vi "New DAQ Rack AI Read.vi"(8 "Rack Version":T2, 9 "Cal Unit":T3, 10 "Channel to Cal":T1, 11 "Chassis":tag) -> (0 "Lost Connection":bool, 2 "Available?":bool, 3 "Data":dbl format="%0.2f")   [LabVIEW 2013]
uses:
  Type Defs/Units Type Def (DAQ Rack).ctl
  Type Defs/Rack Version Type Def.ctl
  Type Defs/New Channel Type Def (RIO).ctl
  Type Defs/TCP Data Stream Mode (PC).ctl
  <vilib>/DAQmx/read.llb/DAQmx Read (Analog DBL 1Chan 1Samp).vi
  <vilib>/DAQmx/read.llb/DAQmx Read (Analog 1D DBL 1Chan NSamp).vi
  <vilib>/DAQmx/create/channels.llb/DAQmx Create Channel (AI-Voltage-Basic).vi
  <vilib>/DAQmx/miscellaneous.llb/DAQmx Fill In Error Info.vi
  <vilib>/DAQmx/configure/timing.llb/DAQmx Timing (Sample Clock).vi
  <resource>/objmgr/daqmx.rc
  <vilib>/DAQmx/create/channels.llb/DAQmx Create Channel (AI-Temperature-Thermocouple).vi
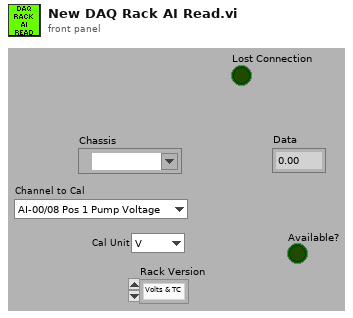
[diagram p1: front panel]
types:
  T1 = typedef "New Channel Type Def (RIO).ctl" = enum16{"AI-00/08 Pos 1 Pump Voltage", "AI-01/09 Pos 2 Pump Voltage", "AI-02/10 Pos 3 Pump Voltage", "AI-03/11 Pos 4 Pump Voltage", "AI-04/12 Pos 5 Pump Voltage", "AI-05/13 Pos 6 Pump Voltage", "AI-06 Spare", "AI-14 Spare", "AI-07 Spare", "AI-15 Power Supply Voltage", "AI-16 Pos 1 Pump Current", "AI-17 Pos 2 Pump Current", "AI-18 Pos 3 Pump Current", "AI-19 Pos 4 Pump Current", "AI-20 Pos 5 Pump Current", "AI-21 Pos 6 Pump Current", "AI-16 Pos 1 Pump Speed", "AI-17 Pos 2 Pump Speed", "AI-18 Pos 3 Pump Speed", "AI-19 Pos 4 Pump Speed", "AI-20 Pos 5 Pump Speed", "AI-21 Pos 6 Pump Speed", "AI-22 Pos 1 Controller Current", "AI-23 Pos 2 Controller Current", "AI-24 Pos 3 Controller Current", "AI-25 Pos 4 Controller Current", "AI-26 Pos 5 Controller Current", "AI-27 Pos 6 Controller Current", "AI-28 Tank 1 Temperature", "AI-29 Tank 2 Temperature", "AI-30 Pos 1 Pump Pressure", "AI-31 Pos 2 Pump Pressure", "AI-32 Pos 3 Pump Pressure", "AI-33 Pos 4 Pump Pressure", "AI-34 Pos 5 Pump Pressure", "AI-35 Pos 6 Pump Pressure", "AI-36 Pos 1 Pump Flow", "AI-37 Pos 2 Pump Flow", "AI-38 Pos 3 Pump Flow", "AI-39 Pos 4 Pump Flow", "AI-40 Pos 5 Pump Flow", "AI-41 Pos 6 Pump Flow", "AI-42 Spare", "AI-43 Spare", "AI-44 Spare", "AI-45 Spare", "AI-46 Spare", "AI-47 Spare", "AI-00/08 Pos 1 Controller Voltage", "AI-01/09 Pos 2 Controller Voltage", "AI-02/10 Pos 3 Controller Voltage", "AI-03/11 Pos 4 Controller Voltage", "AI-04/12 Pos 5 Controller Voltage", "AI-05/13 Pos 6 Controller Voltage"}
  T2 = typedef "Rack Version Type Def.ctl" = enum16{"Volts & TC", "Volts", "RIO", "Volts & Current", "Cart"}
  T3 = typedef "Units Type Def (DAQ Rack).ctl" = enum16{"V", "mA", "A", "Hz", "deg C"}
  T4 = typedef "TCP Data Stream Mode (PC).ctl" = enum16{"Init", "Read Data", "Close"}
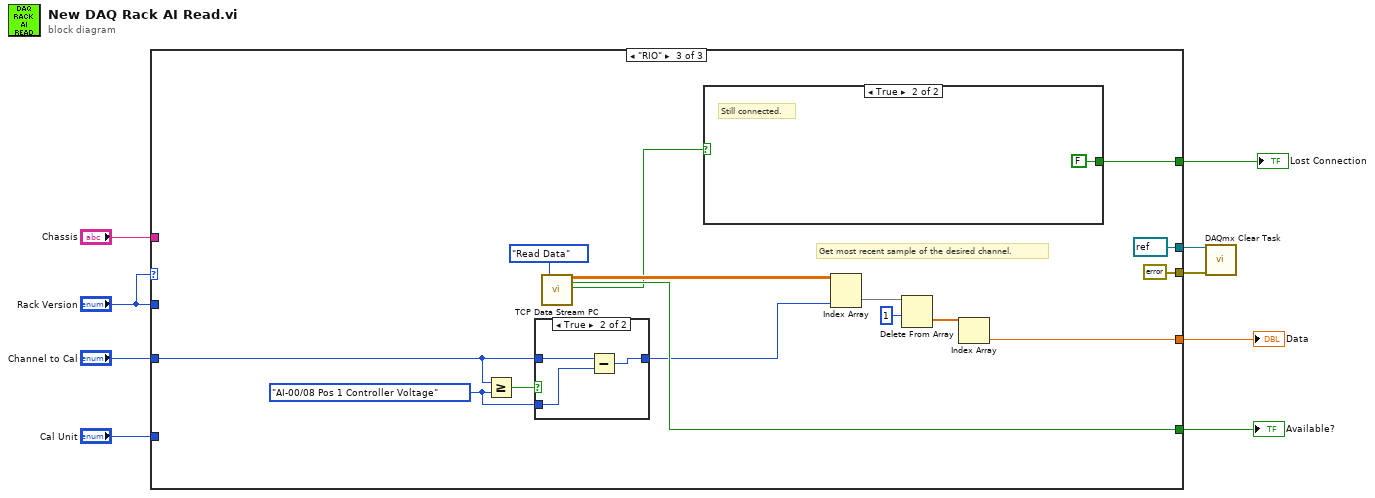
[diagram p0: block diagram]
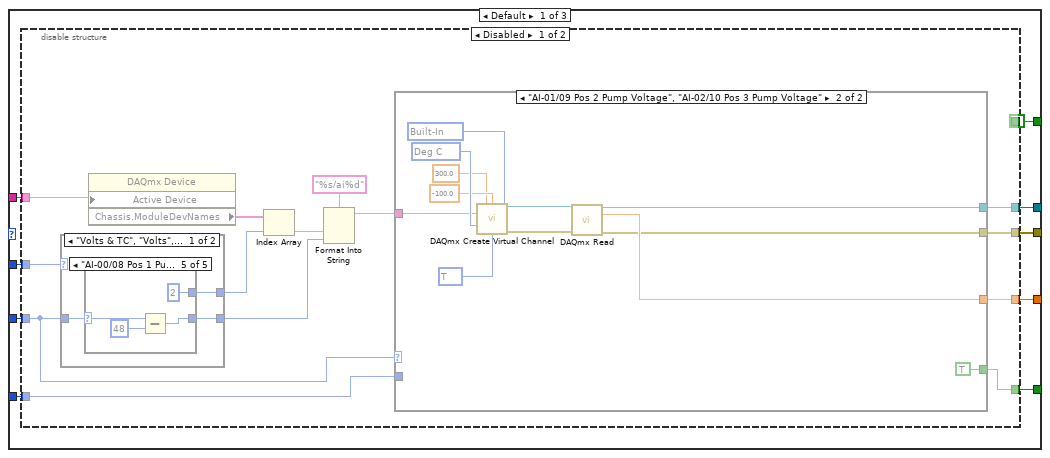
[diagram p2: hidden frame]
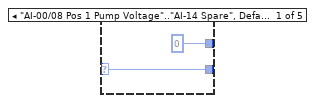
[diagram p3: hidden frame]
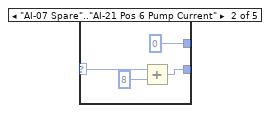
[diagram p4: hidden frame]
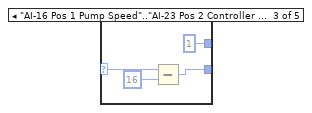
[diagram p5: hidden frame]
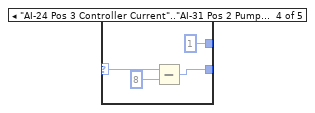
[diagram p6: hidden frame]
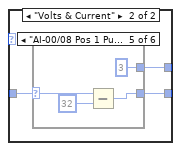
[diagram p7: hidden frame]
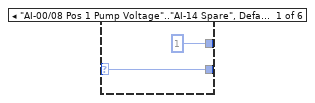
[diagram p8: hidden frame]
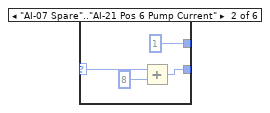
[diagram p9: hidden frame]
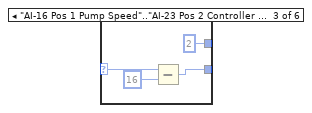
[diagram p10: hidden frame]
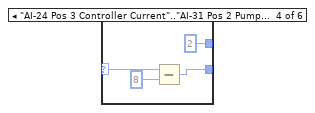
[diagram p11: hidden frame]
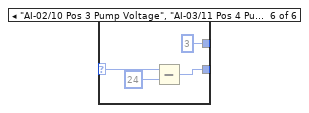
[diagram p12: hidden frame]
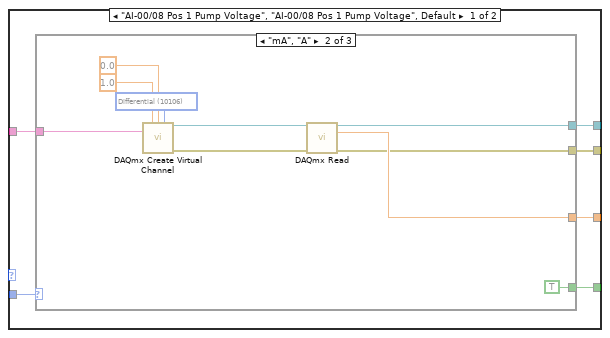
[diagram p13: hidden frame]
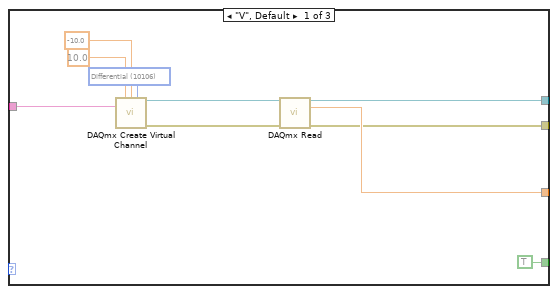
[diagram p14: hidden frame]
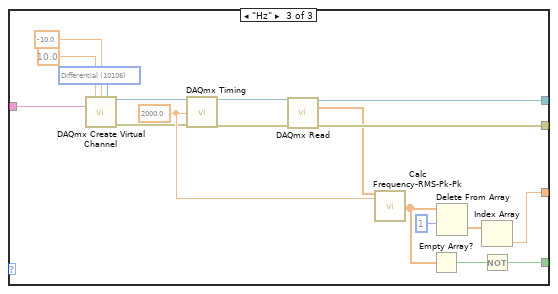
[diagram p15: hidden frame]
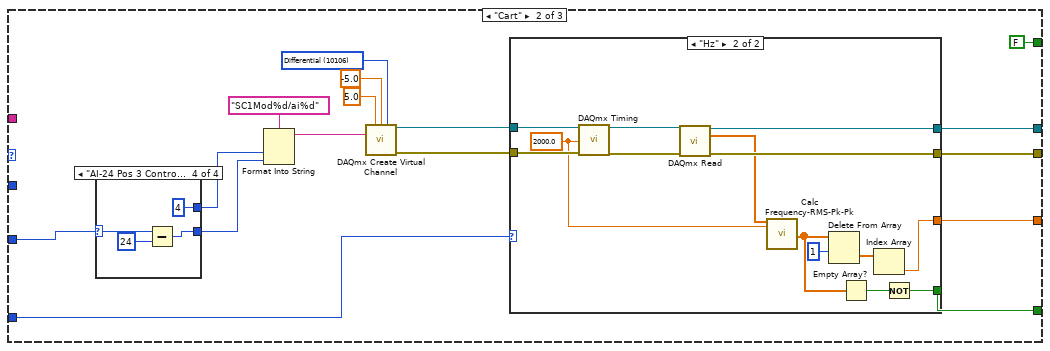
[diagram p17: hidden frame]
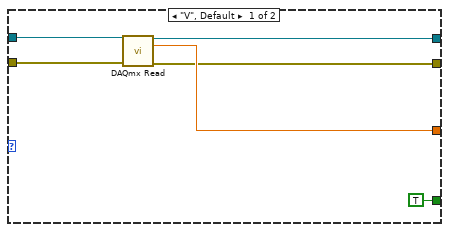
[diagram p18: hidden frame]
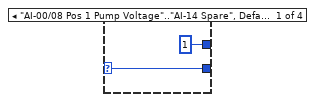
[diagram p19: hidden frame]
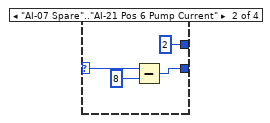
[diagram p20: hidden frame]
diagram:
  n1 = case shown="\"RIO\"" "Rack Version" {
    tunnel: "Channel to Cal" -> [w13 w148 w188]
    tunnel: [w18 w139 w197] -> w9
    tunnel: [w17 w143 refnum<k21> refnum ("task out")] -> w4
    tunnel: [w16 w142 errorcluster {"status"=FALSE, "code"=0, "source"=""} ("error out")] -> w3
    tunnel: "Chassis" -> [w15 _ _]
    tunnel: [w14 w138 w191] -> w7
    tunnel: "Cal Unit" -> [w12 w137 _]
    tunnel: "Rack Version" -> [w11 _ _]
    tunnel: [w10 FALSE w194] -> w2
    frame Default {
      n2 = disable-structure shown="Disabled" {
        disable-tunnel: [w27 _] -> w18
        disable-tunnel: [w26 _] -> w17
        disable-tunnel: [w25 _] -> w16
        disable-tunnel: w15 -> [w24 _]
        disable-tunnel: [w23 _] -> w14
        disable-tunnel: w13 -> [w22 _]
        disable-tunnel: w12 -> [w21 _]
        disable-tunnel: w11 -> [w20 _]
        disable-tunnel: [FALSE _] -> w10
        frame Disabled {
          n3 = case shown="\"Volts & TC\", \"Volts\", Default" w20 {
            tunnel: [w36 w57] -> w32
            tunnel: [w35 w56] -> w29
            tunnel: w22 -> [w34 w55]
            frame "Volts & TC", "Volts", Default {
              n4 = case shown="\"TC-00\"..\"TC-15\"" w34 {
                selector: w34 -> [w37 w40 w45 w49 w52]
                tunnel: [0 ("index") 0 ("index") 1 ("index") 1 ("index") 2 ("index")] -> w36
                tunnel: [w37 w39 w43 w47 w51] -> w35
                frame "AI-00/08 Pos 1 Pump Voltage".."AI-14 Spare", Default {
                }
                frame "AI-07 Spare".."AI-21 Pos 6 Pump Current" {
                  n5 = Add(x=w40, y=u16 8) -> (x+y=w39:u16)
                }
                frame "AI-16 Pos 1 Pump Speed".."AI-23 Pos 2 Controller Current" {
                  n6 = Subtract(x=w45, y=u16 16) -> (x-y=w43:u16)
                }
                frame "AI-24 Pos 3 Controller Current".."AI-31 Pos 2 Pump Pressure" {
                  n7 = Subtract(x=w49, y=u16 8) -> (x-y=w47:u16)
                }
                frame "AI-00/08 Pos 1 Pump Voltage", "AI-01/09 Pos 2 Pump Voltage" {
                  n8 = Subtract(x=w52, y=u16 48) -> (x-y=w51:u16)
                }
              }
            }
            frame "Volts & Current" {
              n9 = case shown="\"AI-32\"..\"AI-39\"" w55 {
                selector: w55 -> [w58 w61 w66 w70 w73 w77]
                tunnel: [1 ("index") 1 ("index") 2 ("index") 2 ("index") 3 ("index") 3 ("index")] -> w57
                tunnel: [w58 w60 w64 w68 w72 w76] -> w56
                frame "AI-00/08 Pos 1 Pump Voltage".."AI-14 Spare", Default {
                }
                frame "AI-07 Spare".."AI-21 Pos 6 Pump Current" {
                  n10 = Add(x=w61, y=u16 8) -> (x+y=w60:u16)
                }
                frame "AI-16 Pos 1 Pump Speed".."AI-23 Pos 2 Controller Current" {
                  n11 = Subtract(x=w66, y=u16 16) -> (x-y=w64:u16)
                }
                frame "AI-24 Pos 3 Controller Current".."AI-31 Pos 2 Pump Pressure" {
                  n12 = Subtract(x=w70, y=u16 8) -> (x-y=w68:u16)
                }
                frame "AI-00/08 Pos 1 Pump Voltage", "AI-01/09 Pos 2 Pump Voltage" {
                  n13 = Subtract(x=w73, y=u16 32) -> (x-y=w72:u16)
                }
                frame "AI-02/10 Pos 3 Pump Voltage", "AI-03/11 Pos 4 Pump Voltage" {
                  n14 = Subtract(x=w77, y=u16 24) -> (x-y=w76:u16)
                }
              }
            }
          }
          n15 = property class="DAQmx Device"("Active Device"=w24) -> ("Chassis.ModuleDevNames"=w33:tag[])  [unwired: 2 in, 2 out]
          n16 = Index Array(array=w33, index=w32) -> (element=w30:tag)
          n17 = Format Into String(format string="%s/ai%d", w30, w29) -> (resulting string=w31:string)  [unwired: 2 in, 1 out]
          n18 = case shown="\"TC-00\"..\"TC-15\"" w22 {
            tunnel: w31 -> [w80 w125]
            tunnel: [w85 w134] -> w27
            tunnel: [w84 w128] -> w26
            tunnel: [w83 w127] -> w25
            tunnel: [w82 TRUE ("empty?")] -> w23
            tunnel: w21 -> [w81 _]
            frame "AI-00/08 Pos 1 Pump Voltage", "AI-00/08 Pos 1 Pump Voltage", Default {
              n19 = case shown="\"mA\", \"A\"" w81 {
                tunnel: [w95 w105 w115] -> w85
                tunnel: [w94 w104 w123] -> w84
                tunnel: [w93 w103 w122] -> w83
                tunnel: [TRUE ("empty?") TRUE ("empty?") w112] -> w82
                tunnel: w80 -> [w86 w96 w106]
                frame "V", Default {
                  w91 = 10106 items=["default"=-1, "RSE"=10083, "NRSE"=10078, "Differential"=10106, "Pseudodifferential"=12529] ("input terminal configuration")
                  n20 = call-poly <vilib>:"DAQmx Create Virtual Channel.vi"("maximum value"=10.0, "minimum value"=-10.0, "input terminal configuration"=w91, "physical channels"=w86) -> ("task out"=w88:refnum<k21>, "error out"=w87:errorcluster)  [unwired: 10 in]
                  n21 = call-poly <vilib>:"DAQmx Read.vi"("task/channels in"=w88, "error in"=w87) -> ("task out"=w94:refnum<k21>, "data"=w95:dbl, "error out"=w93:errorcluster)  [unwired: 11 in]
                }
                frame "mA", "A" {
                  w101 = 10106 items=["default"=-1, "RSE"=10083, "NRSE"=10078, "Differential"=10106, "Pseudodifferential"=12529] ("input terminal configuration")
                  n22 = call-poly <vilib>:"DAQmx Create Virtual Channel.vi"("maximum value"=1.0, "minimum value"=0.0, "input terminal configuration"=w101, "physical channels"=w96) -> ("task out"=w98:refnum<k21>, "error out"=w97:errorcluster)  [unwired: 10 in]
                  n23 = call-poly <vilib>:"DAQmx Read.vi"("task/channels in"=w98, "error in"=w97) -> ("task out"=w104:refnum<k21>, "data"=w105:dbl, "error out"=w103:errorcluster)  [unwired: 11 in]
                }
                frame "Hz" {
                  w111 = 10106 items=["default"=-1, "RSE"=10083, "NRSE"=10078, "Differential"=10106, "Pseudodifferential"=12529] ("input terminal configuration")
                  w118 = 2000.0 ("rate")
                  n24 = call-poly <vilib>:"DAQmx Create Virtual Channel.vi"("maximum value"=10.0, "minimum value"=-10.0, "input terminal configuration"=w111, "physical channels"=w106) -> ("task out"=w107:refnum<k21>, "error out"=w108:errorcluster)  [unwired: 10 in]
                  n25 = call-poly <vilib>:"DAQmx Timing.vi"("task/channels in"=w107, "rate"=w118, "error in"=w108) -> ("task out"=w121:refnum<k21>, "error out"=w120:errorcluster)  [unwired: 11 in]
                  n26 = call-poly <vilib>:"DAQmx Read.vi"("task/channels in"=w121, "error in"=w120) -> ("task out"=w123:refnum<k21>, "data"=w119:dbl[], "error out"=w122:errorcluster)  [unwired: 11 in]
                  n27 = call "Calc Frequency-RMS-Pk-Pk.vi"("Signal Data In"=w119, "Sample Rate"=w118) -> ("Frequency"=w114:dbl[])  [unwired: 13 in, 4 out]
                  n28 = Empty Array?(array=w114) -> (empty?=w113:bool)
                  n29 = Delete From Array(array=w114, length=1) -> (deleted portion=w116:dbl[])  [unwired: 1 in, 1 out]
                  n30 = Index Array(array=w116) -> (element=w115:dbl)  [unwired: 1 in]
                  n31 = Not(x=w113) -> (.not. x?=w112:bool)
                }
              }
            }
            frame "AI-01/09 Pos 2 Pump Voltage", "AI-02/10 Pos 3 Pump Voltage" {
              w126 = 10200 items=["Built-In"=10200, "Constant Value"=10116, "Channel"=10113] ("cjc source")
              w132 = 10143 items=["Deg C"=10143, "Deg F"=10144, "Kelvins"=10325, "Deg R"=10145, "From Custom Scale"=10065] ("units")
              w133 = 10086 items=["J"=10072, "K"=10073, "N"=10077, "R"=10082, "S"=10085, "T"=10086, "B"=10047, "E"=10055] ("thermocouple type")
              n32 = call-poly <vilib>:"DAQmx Create Virtual Channel.vi"("maximum value"=300.0, "minimum value"=-100.0, "physical channels"=w125, "cjc source"=w126, "units"=w132, "thermocouple type"=w133) -> ("task out"=w129:refnum<k21>, "error out"=w135:errorcluster)  [unwired: 8 in]
              n33 = call-poly <vilib>:"DAQmx Read.vi"("task/channels in"=w129, "error in"=w135) -> ("task out"=w128:refnum<k21>, "data"=w134:dbl, "error out"=w127:errorcluster)  [unwired: 11 in]
            }
          }
        }
        frame Enabled {
        }
      }
    }
    frame "Cart" {
      w150 = 10106 items=["default"=-1, "RSE"=10083, "NRSE"=10078, "Differential"=10106, "Pseudodifferential"=12529] ("input terminal configuration")
      n34 = case shown="\"AI-24 Pos 3 Controller Current\"..\"AI-31 Pos 2 Pump Pressure\"" w148 {
        selector: w148 -> [w173 w176 w180 w184]
        tunnel: [w173 w175 w179 w183] -> w146
        tunnel: [u16 1 ("Channel to Cal") u16 2 ("Channel to Cal") u16 3 ("Channel to Cal") u16 4 ("Channel to Cal")] -> w145
        frame "AI-00/08 Pos 1 Pump Voltage".."AI-14 Spare", Default {
        }
        frame "AI-07 Spare".."AI-21 Pos 6 Pump Current" {
          n35 = Subtract(x=w176, y=u16 8) -> (x-y=w175:u16)
        }
        frame "AI-16 Pos 1 Pump Speed".."AI-23 Pos 2 Controller Current" {
          n36 = Subtract(x=w180, y=u16 16) -> (x-y=w179:u16)
        }
        frame "AI-24 Pos 3 Controller Current".."AI-31 Pos 2 Pump Pressure" {
          n37 = Subtract(x=w184, y=u16 24) -> (x-y=w183:u16)
        }
      }
      n38 = Format Into String(format string="SC1Mod%d/ai%d", w145, w146) -> (resulting string=w144:string)  [unwired: 2 in, 1 out]
      n39 = call-poly <vilib>:"DAQmx Create Virtual Channel.vi"("maximum value"=5.0, "minimum value"=-5.0, "input terminal configuration"=w150, "physical channels"=w144) -> ("task out"=w141:refnum<k21>, "error out"=w140:errorcluster)  [unwired: 10 in]
      n40 = case shown="\"Hz\"" w137 {
        tunnel: w141 -> [w157 w169]
        tunnel: w140 -> [w156 w168]
        tunnel: [w155 w161] -> w139
        tunnel: [w154 w171] -> w143
        tunnel: [w153 w170] -> w142
        tunnel: [TRUE ("empty?") w158] -> w138
        frame "V", Default {
          n41 = call-poly <vilib>:"DAQmx Read.vi"("task/channels in"=w157, "error in"=w156) -> ("task out"=w154:refnum<k21>, "data"=w155:dbl, "error out"=w153:errorcluster)  [unwired: 11 in]
        }
        frame "Hz" {
          w164 = 2000.0 ("rate")
          n42 = call-poly <vilib>:"DAQmx Timing.vi"("task/channels in"=w169, "rate"=w164, "error in"=w168) -> ("task out"=w167:refnum<k21>, "error out"=w166:errorcluster)  [unwired: 11 in]
          n43 = call-poly <vilib>:"DAQmx Read.vi"("task/channels in"=w167, "error in"=w166) -> ("task out"=w171:refnum<k21>, "data"=w165:dbl[], "error out"=w170:errorcluster)  [unwired: 11 in]
          n44 = call "Calc Frequency-RMS-Pk-Pk.vi"("Signal Data In"=w165, "Sample Rate"=w164) -> ("Frequency"=w160:dbl[])  [unwired: 13 in, 4 out]
          n45 = Delete From Array(array=w160, length=1) -> (deleted portion=w162:dbl[])  [unwired: 1 in, 1 out]
          n46 = Empty Array?(array=w160) -> (empty?=w159:bool)
          n47 = Index Array(array=w162) -> (element=w161:dbl)  [unwired: 1 in]
          n48 = Not(x=w159) -> (.not. x?=w158:bool)
        }
      }
    }
    frame "RIO" {
      w186 = New_Channel_Type_Def_(RIO)."AI-00/08 Pos 1 Controller Voltage" ("y")
      # "Get most recent sample of the desired channel."
      n49 = Greater Or Equal?(x=w188, y=w186) -> (x >= y?=w189:bool)
      n50 = case shown="True" w189 {
        tunnel: w188 -> [w201 w204]
        tunnel: [w201 w203] -> w187
        tunnel: w186 -> [_ w202]
        frame False {
        }
        frame True {
          n51 = Subtract(x=w204, y=w202) -> (x-y=w203:u16)
        }
      }
      n52 = call "TCP Data Stream PC.vi"("Mode"=TCP_Data_Stream_Mode_(PC)."Read Data") -> ("Data OUT"=w192:dbl[][], "New Data?"=w191:bool, "Connected?"=w190:bool)  [unwired: 15 in, 1 out]
      n53 = case shown="True" w190 {
        tunnel: [TRUE FALSE] -> w194
        frame False {
          # "Lost connection."
          n54 = One Button Dialog(message="Lost connection to network system.\n\nCal is now terminated.") -> ()  [unwired: 1 in, 1 out]
        }
        frame True {
          # "Still connected."
        }
      }
      n55 = Index Array(array=w192, index (col)=w187) -> (element=w200:dbl[])  [unwired: 1 in]
      n56 = Delete From Array(array=w200, length=1) -> (deleted portion=w198:dbl[])  [unwired: 1 in, 1 out]
      n57 = Index Array(array=w198) -> (element=w197:dbl)  [unwired: 1 in]
    }
  }
  "Data" <- w9
  "Available?" <- w7
  "Lost Connection" <- w2
  n58 = call <vilib>:"DAQmx Clear Task.vi"("task in"=w4, "error in"=w3) -> ()  [unwired: 13 in, 1 out]
